vi "Decimate.vi"(6 "Select":enum16{"Pre DSP", "Post DSP"}(ring), 8 "error in (no error)":errorcluster, 11 "Instrument.DAQ":refnum<class "Instrument.DAQ.lvclass">) -> (0 "error out":errorcluster, 3 "Instrument.DAQ out":refnum<class "Instrument.DAQ.lvclass">)   [LabVIEW 2019, in "Instrument.Lockin.lvlib" / "Instrument.DAQ.lvclass"]
doc: "Decimates the input sequence X by the decimating factor and the averaging Boolean control."
uses:
  Instrument.DAQ.lvclass
  Instrument.DAQ.lvclass/Instrument.DAQ.ctl
  DSP/DSP.lvclass
panel:
  out "x-y":dbl
  # "by Marco Tedaldi, Brain Research Institute, University of Zurich, 2013"
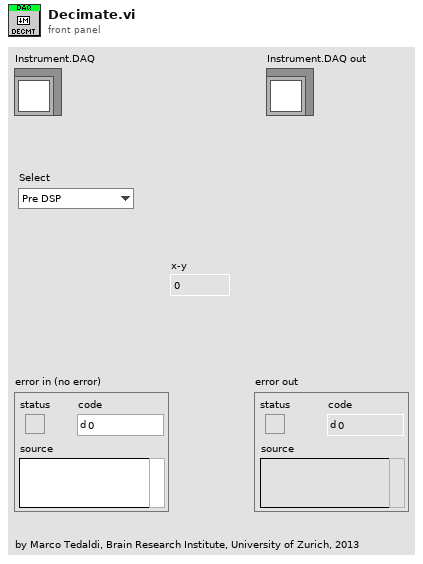
[diagram p1: front panel]
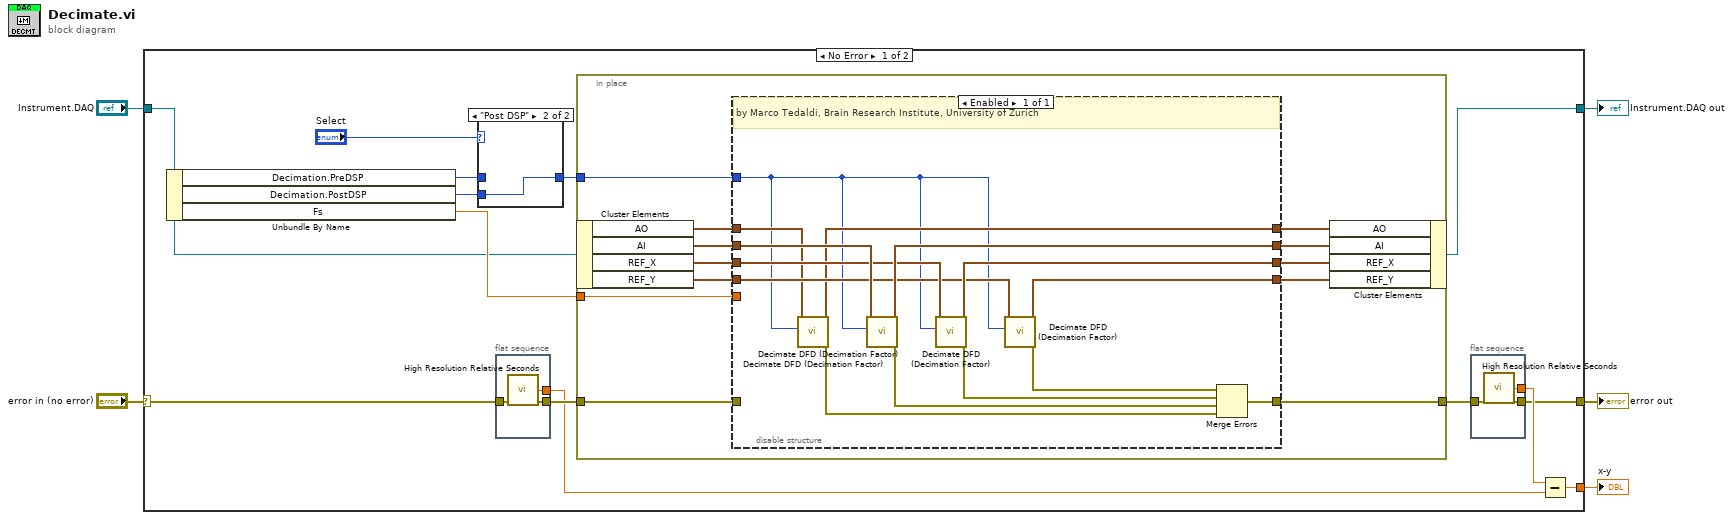
[diagram p0: block diagram]
diagram:
  n1 = case shown="No Error" "error in (no error)" {
    selector: "error in (no error)" -> [w12 w53]
    tunnel: [w8 w53] -> w5
    tunnel: "Instrument.DAQ" -> [w13 w52]
    tunnel: [w14 w52] -> w2
    tunnel: [w7 _] -> w1
    frame No Error {
      n2 = Unbundle By Name(w13) -> ("Decimation.PreDSP"=w17:i32, "Decimation.PostDSP"=w16:i32, "Fs"=w15:dbl)
      n3 = case shown="\"Post DSP\"" "Select" {
        tunnel: [w24 w25] -> w18
        tunnel: w17 -> [w24 _]
        tunnel: w16 -> [_ w25]
        frame "Pre DSP", Default {
        }
        frame "Post DSP" {
        }
      }
      n4 = flat-sequence {
        tunnel: [w23] -> w11
        tunnel: w12 -> [w23]
        tunnel: [w22] -> w6
        frame #0 {
          n5 = call <vilib>:"High Resolution Relative Seconds.vi"() -> ("relative seconds"=w22:dbl)
        }
      }
      n6 = in-place {
        in-place-border: [w26] -> w9
        in-place-border: w18 -> [w37]
        in-place-border: w15 -> [w33]
        in-place-border: w11 -> [w27]
        n7 = in-place-cluster #1(w13) -> ("AO"=w36:waveform(dbl)[], "AI"=w35:waveform(dbl)[], "REF_X"=w34:waveform(dbl)[], "REF_Y"=w32:waveform(dbl)[])
        n8 = disable-structure shown="Enabled" {
          disable-tunnel: w27 -> [_]
          disable-tunnel: [w39] -> w31
          disable-tunnel: [w45] -> w26
          disable-tunnel: w36 -> [w40]
          disable-tunnel: w37 -> [w38]
          disable-tunnel: w33 -> [_]
          disable-tunnel: w35 -> [w51]
          disable-tunnel: [w50] -> w30
          disable-tunnel: w34 -> [w49]
          disable-tunnel: [w48] -> w29
          disable-tunnel: w32 -> [w47]
          disable-tunnel: [w46] -> w28
          frame Enabled {
            # "by Marco Tedaldi, Brain Research Institute, University of Zurich"
            n9 = call "Decimate DFD (Decimation Factor).vi"("Decimation Factor"=w38, "Waveforms in"=w40) -> ("error out"=w41:errorcluster, "waveforms out"=w39:waveform(dbl)[])  [unwired: 8 in]
            n10 = call "Decimate DFD (Decimation Factor).vi"("Decimation Factor"=w38, "Waveforms in"=w51) -> ("error out"=w42:errorcluster, "waveforms out"=w50:waveform(dbl)[])  [unwired: 8 in]
            n11 = call "Decimate DFD (Decimation Factor).vi"("Decimation Factor"=w38, "Waveforms in"=w49) -> ("error out"=w43:errorcluster, "waveforms out"=w48:waveform(dbl)[])  [unwired: 8 in]
            n12 = call "Decimate DFD (Decimation Factor).vi"("Decimation Factor"=w38, "Waveforms in"=w47) -> ("error out"=w44:errorcluster, "waveforms out"=w46:waveform(dbl)[])  [unwired: 8 in]
            n13 = Merge Errors(w44, w43, w42, w41) -> (w45:errorcluster)
          }
        }
        n14 = in-place-cluster #1("AO"=w31, "AI"=w30, "REF_X"=w29, "REF_Y"=w28) -> (w14:refnum<class "Instrument.DAQ.lvclass">)
      }
      n15 = flat-sequence {
        tunnel: [w21] -> w8
        tunnel: w9 -> [w21]
        tunnel: [w20] -> w10
        frame #0 {
          n16 = call <vilib>:"High Resolution Relative Seconds.vi"() -> ("relative seconds"=w20:dbl)
        }
      }
      n17 = Subtract(x=w10, y=w6) -> (x-y=w7:dbl)
    }
    frame Error {
    }
  }
  "error out" <- w5
  "Instrument.DAQ out" <- w2
  "x-y" <- w1
